vi "Configure.vi"(8 "error in (no error)":errorcluster) -> (0 "error out":errorcluster, 1 "valid config":bool, 3 "config":T1)   [LabVIEW 2017, in "McsaOpState.lvlib"]
uses:
  <vilib>/addons/InsightCM/Devices/Shared/Mcsa/McsaOpState/McsaOpState.lvlib
  <vilib>/addons/InsightCM/Devices/Shared/Common/OpState/controls/config.ctl
  <vilib>/addons/InsightCM/Utilities/GlobalConfiguration/GlobalConfiguration.lvlib
  <vilib>/addons/InsightCM/Devices/Shared/Common/OpState/OpState.lvlib
  <vilib>/addons/InsightCM/Devices/Shared/Mcsa/McsaVirtualChannel/McsaVirtualChannel.lvlib
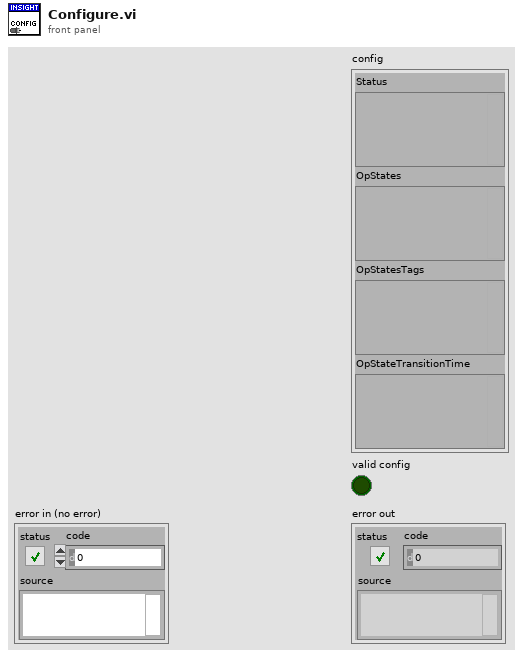
[diagram p1: front panel]
types:
  T1 = typedef "OpState.lvlib/config.ctl" = cluster{"Status":variant, "OpStates":variant, "OpStatesTags":variant, "OpStateTransitionTime":variant}
  T2 = typedef "R2_Device.ctl" = cluster{"Id":string, "Name":string, "DeviceType":string, "HardwareName":string, "IpAddress":string, "HardwareInfo":T3[], "ApplicationType":string, "ApplicationVersion":string, "EquipmentIds":string[], "ConfigurationVersion":string, "State":T4, "Properties":T3[], "DataGroups":T5[], "BurstModeTrigger":T9}
  T3 = typedef "KeyValuePair.ctl" = cluster{"Key":string, "Value":string}
  T4 = typedef "DeviceState.ctl" = cluster{"Disabled":bool}
  T5 = typedef "R2_DataGroup.ctl" = cluster{"Name":string, "OperatingStates":T6[], "Properties":T3[], "EquipmentIds":string[], "AssetNodeId":string}
  T6 = typedef "OperatingState.ctl" = cluster{"Name":string, "Properties":T3[], "Triggers":T7[]}
  T7 = typedef "Trigger.ctl" = cluster{"Type":string, "Expression":string, "Conditions":T8[]}
  T8 = typedef "Condition.ctl" = cluster{"Source":string, "Type":string, "Operator":string, "CompareTo":string, "DwellSeconds":dbl}
  T9 = typedef "BurstModeTrigger.ctl" = cluster{"Trigger":T7, "SampleRate":string, "AcquisitionLength":string}
  T10 = typedef "ConfigListItem.ctl" = cluster{"Id":string, "Name":string, "ReadOnly":bool, "Weight":i32}
  T11 = typedef "MetricDefinitionInstance.ctl" = cluster{"Id":string, "MetricType":string, "Name":string, "Properties":T3[], "HighRate":bool}
  T12 = typedef "SectionKeyValues.ctl" = cluster{"Section":string, "KeyValues":T3[]}
  T13 = typedef "AssetNode.ctl" = cluster{"Id":string, "Type":string, "Name":string, "ParentIds":string[], "State":T14, "MeasType":string, "Properties":T3[], "OperatingStates":T6[], "Metrics":T15[], "TrendAlarmRules":T16[], "References":T19[]}
  T14 = typedef "AssetState.ctl" = cluster{"Disabled":bool}
  T15 = typedef "Metric.ctl" = cluster{"Id":string, "Name":string, "Unit":string, "Properties":T3[], "MetricDefinitionInstanceId":string}
  T16 = typedef "TrendAlarmRule.ctl" = cluster{"Id":string, "AssetNodeId":string, "TrendId":string, "Disabled":bool, "OperatingState":string, "Operator":string, "Hysteresis":dbl, "OnDelaySeconds":dbl, "OffDelaySeconds":dbl, "Levels":T17[], "Properties":T3[]}
  T17 = typedef "TrendAlarmLevel.ctl" = cluster{"Severity":i32, "CompareTo":dbl, "Actions":T18[]}
  T18 = typedef "AlarmAction.ctl" = cluster{"Type":string, "Props":T3[]}
  T19 = typedef "AssetNodeReference.ctl" = cluster{"NodeId":string, "Name":string}
  T20 = typedef "R2_Channel.ctl" = cluster{"Id":string, "DeviceId":string, "Name":string, "ChannelType":string, "HardwareKey":string, "HardwareChannel":string, "DataGroup":string, "Keywords":string[], "EquipmentIds":string[], "Properties":T3[], "Metrics":T15[], "AssetNodeId":string, "MeasType":string, "AssetName":string}
  T21 = typedef "Tag.ctl" = cluster{"Id":string, "Path":string, "Name":string, "Datatype":string, "Props":T3[], "Keywords":string[]}
  T22 = typedef "OpState.lvlib/TriggerOperatingState.ctl" = cluster{"Id":string, "Name":string, "Properties":T3[], "EnterExpression":string, "EnterConditions":T23[], "ExitExpression":string, "ExitConditions":T23[]}
  T23 = typedef "Trigger.lvlib/TriggerCondition.ctl" = cluster{"Condition":T8, "LatchValue":string, "LatchTime":timestamp}
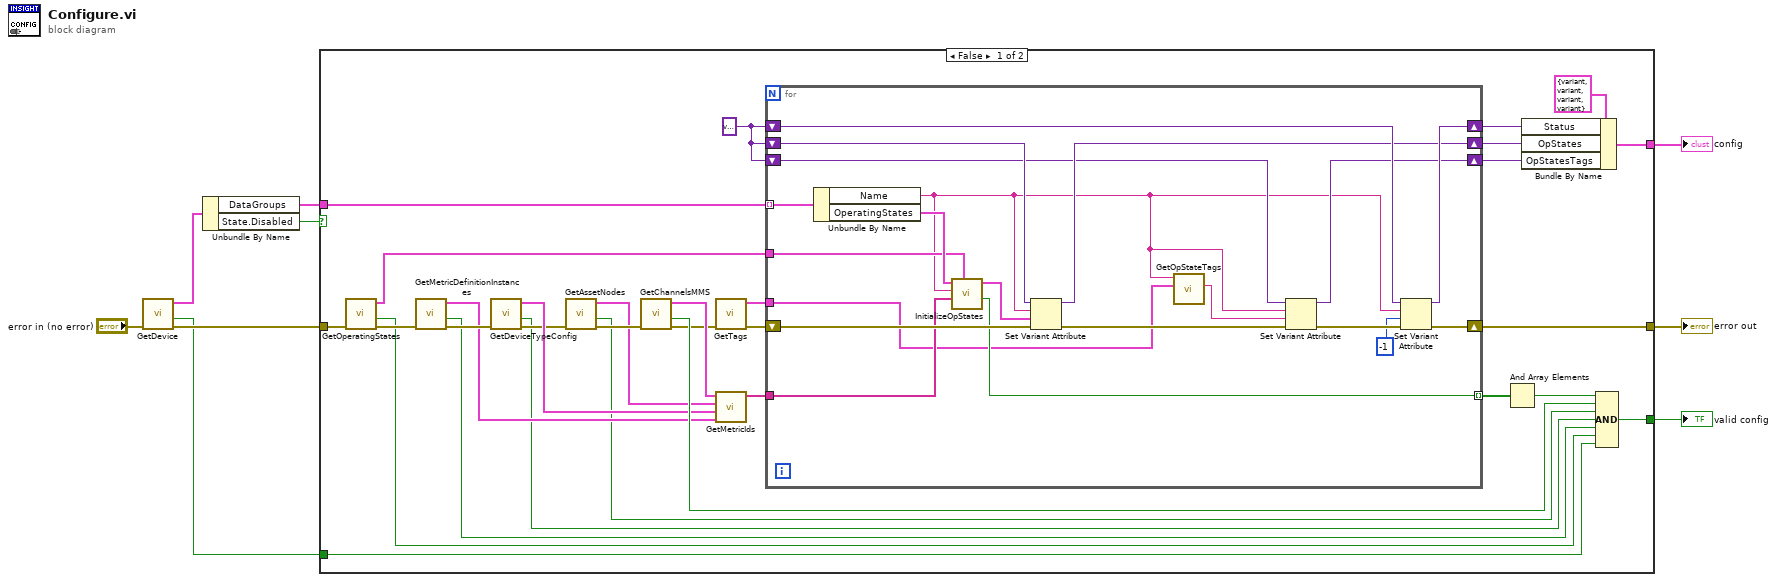
[diagram p0: block diagram]
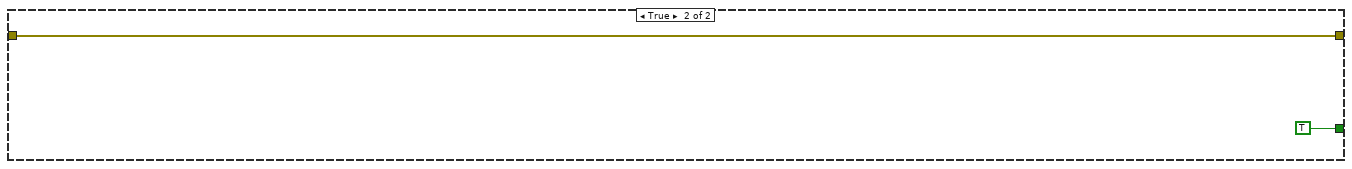
[diagram p2: hidden frame]
diagram:
  n1 = call <vilib>:"GetDevice.vi"("error in (no error)"="error in (no error)") -> ("error out"=w3:errorcluster, "found"=w2:bool, "device configuration"=w8:T2)  [unwired: 8 in]
  n2 = Unbundle By Name(w8) -> ("DataGroups"=w7:T5[], "State.Disabled"=w1:bool)
  n3 = case shown="False" w1 {
    tunnel: w7 -> [w40 _]
    tunnel: [w39 w61] -> w6
    tunnel: [w35 _] -> w5
    tunnel: [w26 TRUE] -> w4
    tunnel: w3 -> [w14 w61]
    tunnel: w2 -> [w12 _]
    frame False {
      w32 = variant ("Status")
      n4 = call <vilib>:"GetOperatingStates.vi"("error in (no error)"=w14) -> ("error out"=w13:errorcluster, "found"=w11:bool, "OperatingStates"=w10:T10[])  [unwired: 8 in]
      n5 = call <vilib>:"GetMetricDefinitionInstances.vi"("error in (no error)"=w13) -> ("error out"=w22:errorcluster, "found"=w15:bool, "metrics"=w18:T11[])  [unwired: 8 in]
      n6 = call <vilib>:"GetDeviceTypeConfig.vi"("error in (no error)"=w22) -> ("error out"=w21:errorcluster, "found"=w16:bool, "key values"=w23:T12[])  [unwired: 8 in]
      n7 = call <vilib>:"GetAssetNodes.vi"("error in (no error)"=w21) -> ("error out"=w20:errorcluster, "found"=w17:bool, "AssetNodes"=w19:T13[])  [unwired: 8 in]
      n8 = call <vilib>:"GetChannelsMMS.vi"("error in (no error)"=w20) -> ("error out"=w24:errorcluster, "found"=w25:bool, "MMS Channels"=w30:T20[])  [unwired: 6 in, 2 out]
      n9 = call <vilib>:"GetTags.vi"("error in (no error)"=w24) -> ("error out"=w34:errorcluster, "tags"=w31:T21[])  [unwired: 8 in, 1 out]
      n10 = call <vilib>:"GetMetricIds.vi"("metrics"=w18, "device type config"=w23, "AssetNodes"=w19, "channels"=w30) -> ("metric ids"=w29:string[])  [unwired: 7 in]
      n11 = for {
        tunnel: w40 -> [w60] mode=indexing
        shift-right: [w57] -> w38
        shift-left: w32 -> [w58]
        shift-right: [w55] -> w37
        shift-left: w32 -> [w59]
        shift-right: [w48] -> w39
        shift-left: w34 -> [w49]
        shift-right: [w51] -> w33
        shift-left: w32 -> [w52]
        tunnel: w31 -> [w42]
        tunnel: w29 -> [w46]
        tunnel: [w45] -> w28 mode=indexing
        tunnel: w10 -> [w44]
        n12 = Unbundle By Name(w60) -> ("Name"=w41:string, "OperatingStates"=w50:T6[])
        n13 = call <vilib>:"InitializeOpStates.vi"("op state defs"=w44, "metric ids"=w46, "data group name"=w41, "operating states in"=w50) -> ("valid config"=w45:bool, "sorted operating states"=w56:T22[])  [unwired: 6 in]
        n14 = Set Variant Attribute(Variant=w59, name=w41, value=w56, error in=w49) -> (Variant out=w55:variant, error out=w54:errorcluster)  [unwired: 1 out]
        n15 = call <vilib>:"GetOpStateTags.vi"("tags"=w42, "data group"=w41) -> ("op state tag id"=w43:string)  [unwired: 9 in]
        n16 = Set Variant Attribute(Variant=w52, name=w41, value=w43, error in=w54) -> (Variant out=w51:variant, error out=w53:errorcluster)  [unwired: 1 out]
        n17 = Set Variant Attribute(Variant=w58, name=w41, value=-1 ("CurrentOpState"), error in=w53) -> (Variant out=w57:variant, error out=w48:errorcluster)  [unwired: 1 out]
      }
      n18 = And Array Elements(Boolean array=w28) -> (logical AND=w27:bool)
      n19 = Bundle By Name(cluster=T1 {"Status"=variant, "OpStates"=variant, "OpStatesTags"=variant, "OpStateTransitionTime"=variant} ("config"), "Status"=w38, "OpStates"=w37, "OpStatesTags"=w33) -> (w35:T1)
      n20 = Compound Arithmetic op=AND(w27, w25, w17, w16, w15, w11, w12) -> (w26:bool)
    }
    frame True {
    }
  }
  "error out" <- w6
  "config" <- w5
  "valid config" <- w4
